vi "Initialize Request Response Queues.vi"(8 "error in (no error)":errorcluster, 9 "Response Queue in":refnum<class "Abstract Message Queue.lvclass">, 10 "Request Queue in":refnum<class "Abstract Message Queue.lvclass">, 11 "Name":string) -> (0 "error out":errorcluster, 1 "Response Queue out":refnum<class "Abstract Message Queue.lvclass">, 2 "Request Queue out":refnum<class "Abstract Message Queue.lvclass">)   [LabVIEW 2017, in "Messaging.lvlib"]
uses:
  Messaging.lvlib
  Message Queue/Abstract Message Queue/Abstract Message Queue.lvclass
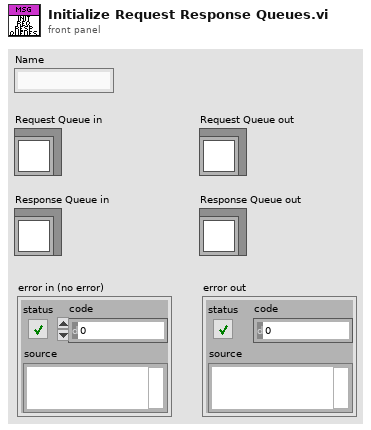
[diagram p1: front panel]
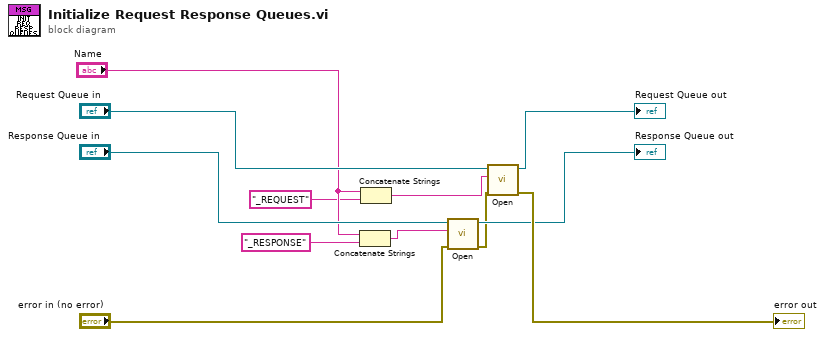
[diagram p0: block diagram]
diagram:
  n1 = Concatenate Strings("Name", "_RESPONSE" ("string")) -> (w7:string)
  n2 = Concatenate Strings("Name", "_REQUEST" ("string")) -> (w5:string)
  n3 = call-dynamic "Open.vi"("error in (no error)"="error in (no error)", "name (unnamed)"=w7, "Abstract Message Queue in"="Response Queue in") -> ("error out"=w2:errorcluster, "Abstract Message Queue out"=→"Response Queue out":refnum<class "Abstract Message Queue.lvclass">)  [unwired: 7 in]
  n4 = call-dynamic "Open.vi"("error in (no error)"=w2, "name (unnamed)"=w5, "Abstract Message Queue in"="Request Queue in") -> ("error out"=→"error out":errorcluster, "Abstract Message Queue out"=→"Request Queue out":refnum<class "Abstract Message Queue.lvclass">)  [unwired: 7 in]
